vi "LS370 Change Excitation Com.vi"(1 "command text in":string[](array[string]), 2 "option":T2) -> (0 "Command text out":string[][](array[string]))   [LabVIEW 2024]
uses:
  LS370 Excitation Voltage.ctl
  LS370 Resistance Range.ctl
  Ctl/option.ctl
  LS370 Excitation Current.ctl
panel:
  in  "Current":T1
  in  "Mode":enum32{"Voltage", "Current"}(radio)
  in  "VISA Resource Name":refnum<visa-resource-name> caption="VISA Name"
  in  "Resistance Range":T3
  in  "enter":bool
  in  "extra wait":i32 min=0
  in  "Channel":i32=1 min=1 max=16 step=1
  in  "Voltage":T4
  in  "cancel":bool
  # "seconds"
  # "AND wait extra"
  # "LakeShore 370 Change Excitation"
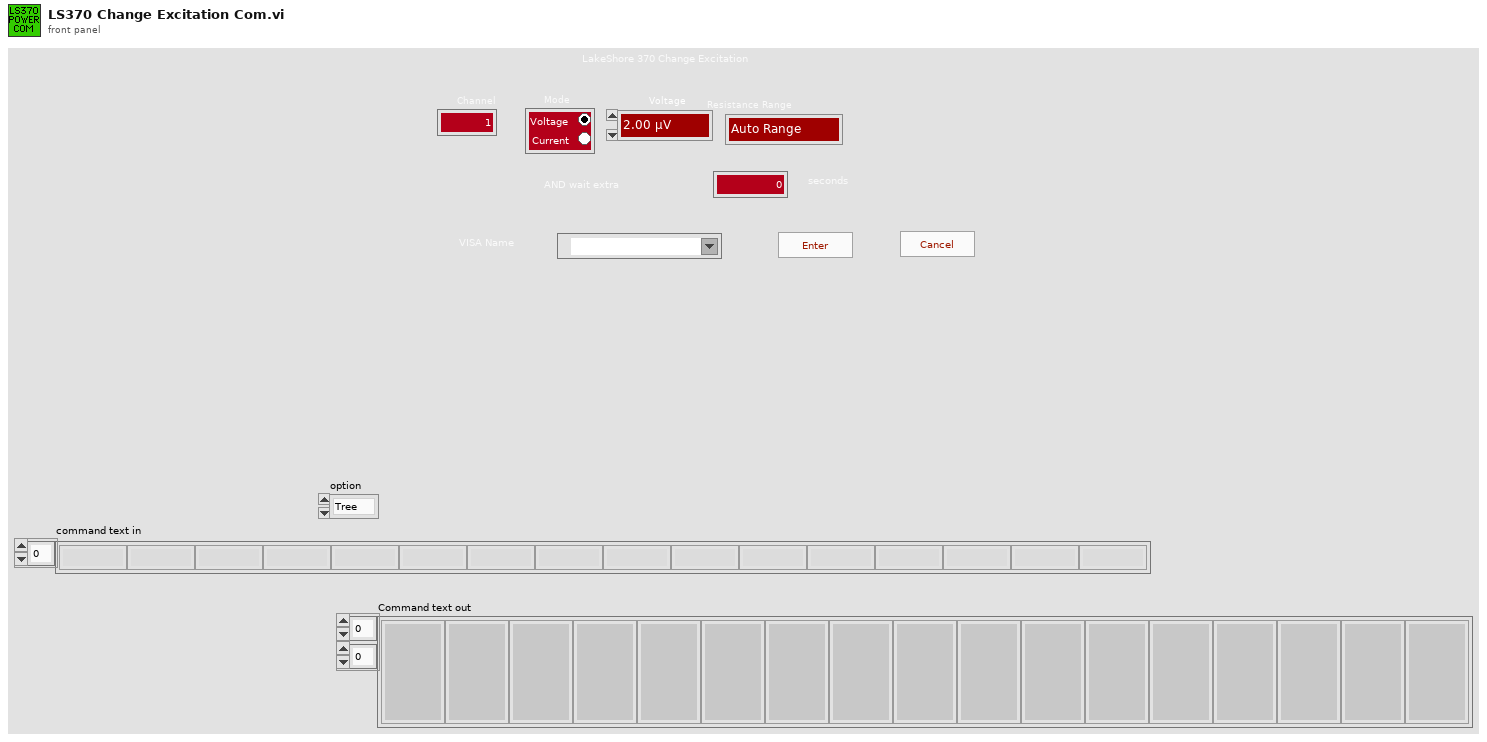
[diagram p1: front panel]
types:
  T1 = typedef "LS370 Excitation Current.ctl" = enum16{"1.00 pA", "3.16 pA", "10.0 pA", "31.6 pA", "100 pA", "316 pA", "1.00 nA", "3.16 nA", "10.0 nA", "31.6 nA", "100 nA", "316 nA", "1.00 µA", "3.16 µA", "10.0 µA", "31.6 µA", "100 µA", "316 µA", "1.00 mA", "3.16mA", "10.0 mA", "31.6 mA"}
  T2 = typedef "option.ctl" = enum16{"Tree", "List"}
  T3 = typedef "LS370 Resistance Range.ctl" = enum16{"Auto Range", "2.00 mΩ", "6.32 mΩ", "20.0 mΩ", "63.2 mΩ", "200 mΩ", "632 mΩ", "2.00 Ω", "6.32 Ω", "20.0 Ω", "63.2 Ω", "200 Ω", "632 Ω", "2.00 kΩ", "6.32 kΩ", "20.0 kΩ", "63.2 kΩ", "200 kΩ", "632 kΩ", "2.00 MΩ", "6.32 MΩ", "20.0 MΩ", "63.2 MΩ"}
  T4 = typedef "LS370 Excitation Voltage.ctl" = enum16{"2.00 µV", "6.32 µV", "20.0 µV", "63.2 µV", "200 µV", "632 µV", "2.00 mV", "6.32 mV", "20.0 mV", "63.2 mV", "200 mV", "632 mV"}
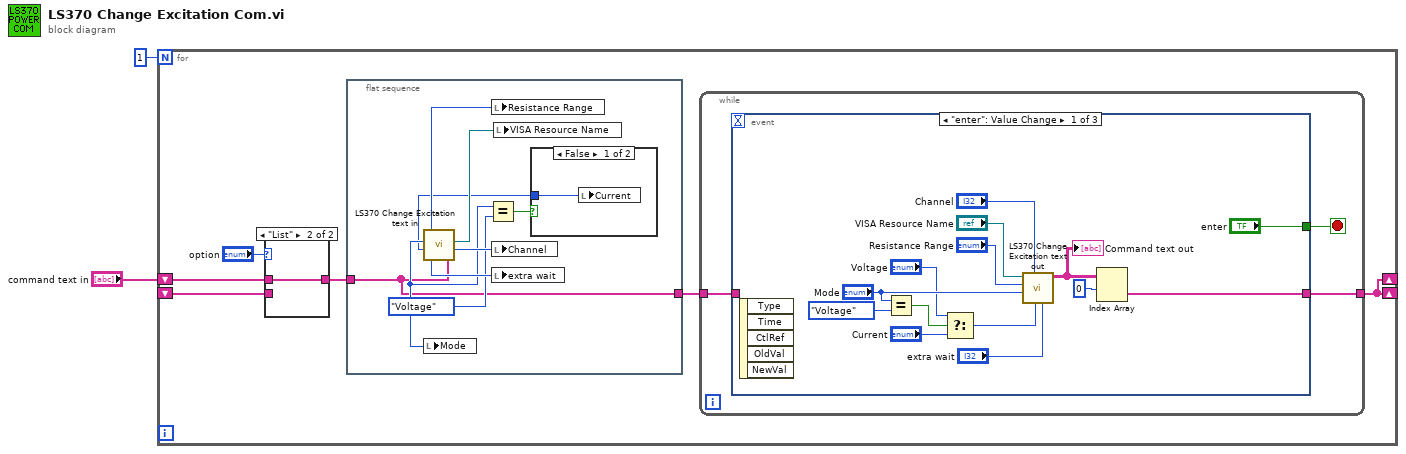
[diagram p0: block diagram]
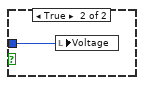
[diagram p2: hidden frame]
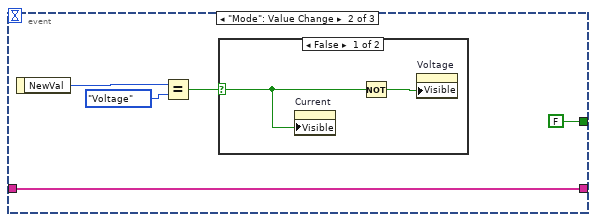
[diagram p3: hidden frame]
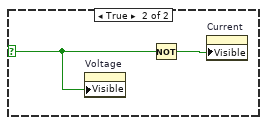
[diagram p4: hidden frame]
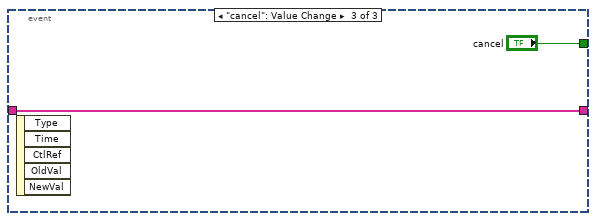
[diagram p5: hidden frame]
diagram:
  n1 = for {
    N: 1 -> [_]
    shift-right: [w5] -> _
    shift-left: _ -> [w6]
    shift-right: [w5] -> _
    shift-left: "command text in" -> [w7]
    n2 = case shown="\"List\"" "option" {
      tunnel: [w48 w49] -> w4
      tunnel: w6 -> [w48 _]
      tunnel: w7 -> [_ w49]
      frame "Tree", Default {
      }
      frame "List" {
      }
    }
    n3 = flat-sequence {
      tunnel: w4 -> [w9]
      tunnel: [w9] -> w3
      frame #0 {
        n4 = call "LS370 Change Excitation text in.vi"("command text in"=w9) -> ("Channel"=w15:i32, "VISA Refnum in"=w17:refnum<visa-resource-name>, "extra wait"=w16:i32, "Current"=w10:u16, "Mode"=w14:enum32{"Voltage", "Current"}, "Resistance Range"=w12:T3)  [unwired: 1 out]
        n5 = local write "Mode"(w14) -> ()
        n6 = Equal?(x=w14, y=enum32{"Voltage", "Current"}."Voltage") -> (x = y?=w11:bool)
        n7 = local write "Resistance Range"(w12) -> ()
        n8 = local write "Channel"(w15) -> ()
        n9 = local write "extra wait"(w16) -> ()
        n10 = local write "VISA Resource Name"(w17) -> ()
        n11 = case shown="False" w11 {
          tunnel: w10 -> [w18 w19]
          frame False {
            n12 = local write "Current"(w18) -> ()
          }
          frame True {
            n13 = local write "Voltage"(w19) -> ()
          }
        }
      }
    }
    n14 = while {
      tunnel: [w21] -> w5
      tunnel: w3 -> [w20]
      stop <- w22 stop-if-true
      n15 = event shown="[0] \"enter\": Value Change" {
        selector: _ -> [_ _ _]
        dyn-events: _ -> [_ _ _]
        timeout: _ -> [_ _ _]
        tunnel: ["enter" FALSE ("cancel") "cancel"] -> w22
        tunnel: [w29 w38 w46] -> w21
        tunnel: w20 -> [_ w38 w46]
        event "enter": Value Change {
          n16 = event-data() -> ()  [unwired: 1 in, 5 out]
          n17 = Equal?(x="Mode", y=enum32{"Voltage", "Current"}."Voltage") -> (x = y?=w27:bool)
          n18 = Select(t="Voltage", s=w27, f="Current") -> (s? t:f=w26:u16)
          n19 = call "LS370 Change Excitation text out.vi"("extra wait"="extra wait", "Current"=w26, "Channel"="Channel", "Mode"="Mode", "Resistance Range"="Resistance Range", "VISA Refnum in"="VISA Resource Name") -> ("Command text"=w33:string[][])  [unwired: 5 in]
          "Command text out" <- w33
          n20 = Index Array(array=w33, index (row)=0) -> (element=w29:string[])  [unwired: 1 in]
        }
        event "Mode": Value Change {
          n21 = event-data() -> ("NewVal"=w41:enum32{"Voltage", "Current"})  [unwired: 1 in]
          n22 = Equal?(x=w41, y=enum32{"Voltage", "Current"}."Voltage") -> (x = y?=w39:bool)
          n23 = case shown="False" w39 {
            selector: w39 -> [w42 w45]
            frame False {
              n24 = property on="Current" class="Enum (strict)"("Visible"=w42) -> ()  [unwired: 2 in, 2 out]
              n25 = Not(x=w42) -> (.not. x?=w43:bool)
              n26 = property on="Voltage" class="Enum (strict)"("Visible"=w43) -> ()  [unwired: 2 in, 2 out]
            }
            frame True {
              n27 = property on="Voltage" class="Enum (strict)"("Visible"=w45) -> ()  [unwired: 2 in, 2 out]
              n28 = Not(x=w45) -> (.not. x?=w44:bool)
              n29 = property on="Current" class="Enum (strict)"("Visible"=w44) -> ()  [unwired: 2 in, 2 out]
            }
          }
        }
        event "cancel": Value Change {
          n30 = event-data() -> ()  [unwired: 1 in, 5 out]
        }
      }
    }
  }
